vi "acquisitionGetFrame.vi"(1 "index":i32, 2 "hamamatsuFrameReferences":refnum<data-value>[](array[refnum])) -> (0 "frameOut":u16[][](array[numeric]))   [LabVIEW 2017]
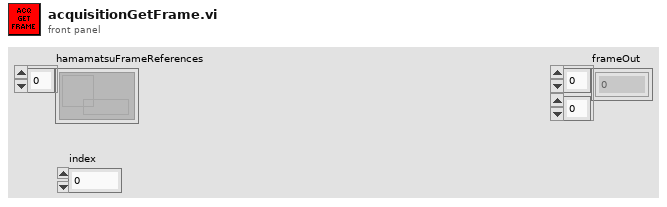
[diagram p1: front panel]
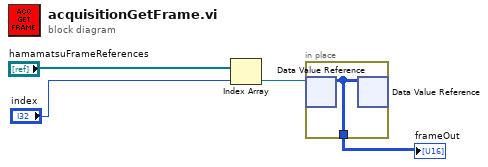
[diagram p0: block diagram]
diagram:
  n1 = Index Array(array="hamamatsuFrameReferences", index="index") -> (element=w2:refnum<data-value>)
  n2 = in-place {
    in-place-border: [w5] -> w1
    n3 = in-place-dvr #1(w2) -> (w5:u16[][])  [unwired: 1 out]
    n4 = in-place-dvr #1(w5) -> ()  [unwired: 2 out]
  }
  "frameOut" <- w1
